vi "Circular.vi"(5 "Direction":u16(ring) items=["Clockwise", "Counter-clockwise"], 6 "return immediately":bool, 7 "Speed":dbl, 8 "error in (no error)":errorcluster, 9 "XY End":dbl[](array[numeric]), 10 "XY Center":dbl[](array[numeric]), 11 "Gantry":refnum<k24>) -> (0 "error IO":errorcluster, 3 "Gantry  2":refnum<k24>)   [LabVIEW 2020, in "Motion.lvclass"]
uses:
  Motion.lvclass
  C:/Program Files (x86)/Aerotech/A3200/LabVIEW/2010/Bin/Aerotech.A3200.dll
  Program Files (x86)/Aerotech/A3200/LabVIEW/2010/Bin/Aerotech.A3200.dll
  Drivers/Aerotech A3200/Motion/CircularCenter.vi
  Drivers/Aerotech A3200/Aerotech.lvlib
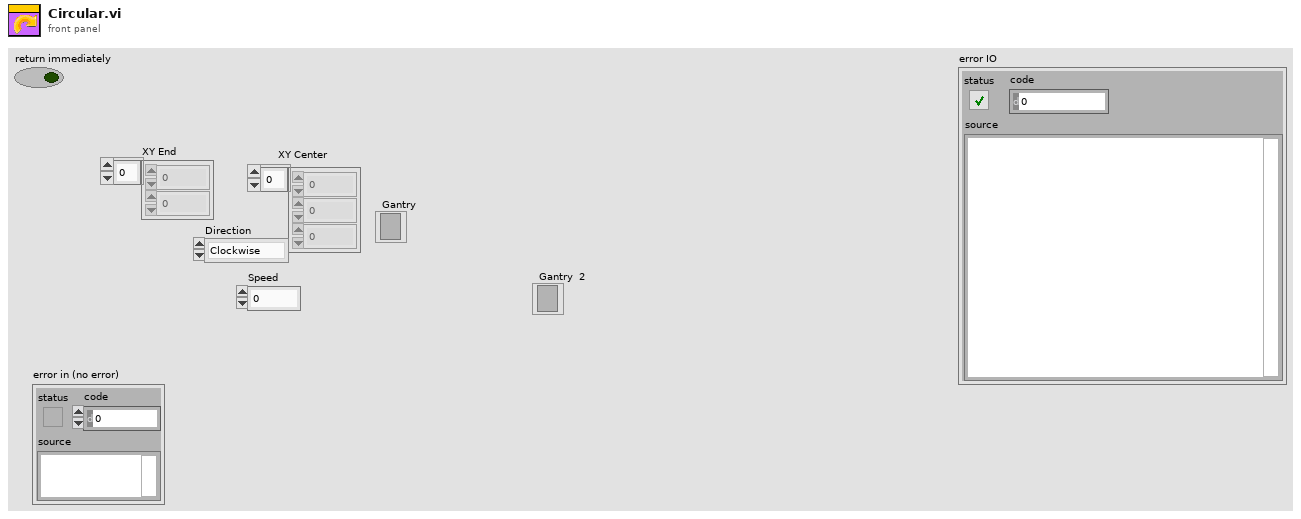
[diagram p1: front panel]
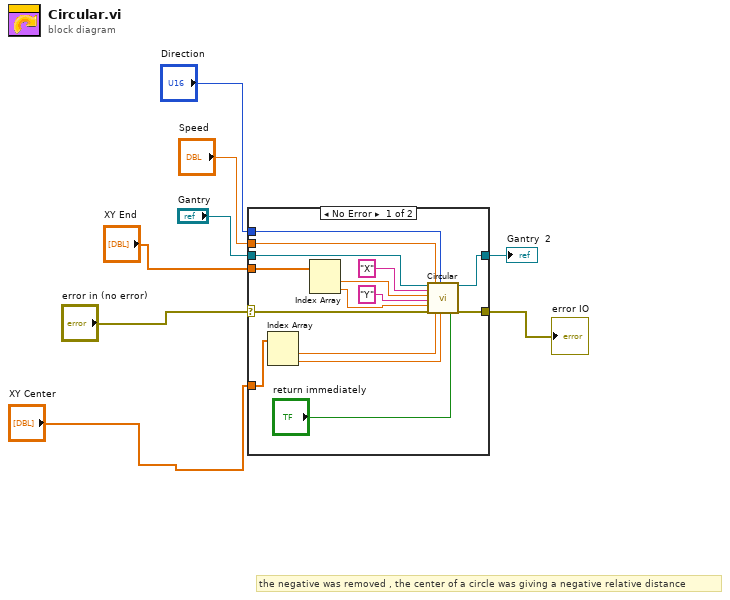
[diagram p0: block diagram]
diagram:
  # "the negative was removed , the center of a circle was giving a negative relative distance"
  n1 = case shown="No Error" "error in (no error)" {
    selector: "error in (no error)" -> [w17 w24]
    tunnel: "XY Center" -> [w22 _]
    tunnel: "Speed" -> [w16 _]
    tunnel: "Direction" -> [w23 _]
    tunnel: [w20 w25] -> w6
    tunnel: "Gantry" -> [w19 w25]
    tunnel: [w18 w24] -> w4
    tunnel: "XY End" -> [w9 _]
    frame No Error {
      n2 = Index Array(array=w22) -> (element #1=w11:dbl, element #2=w10:dbl)  [unwired: 2 in]
      n3 = Index Array(array=w9) -> (element #1=w14:dbl, element #2=w12:dbl)  [unwired: 2 in]
      n4 = call-poly "Circular.vi"("controller in"=w19, "axis 1 name"="X", "axis 1 endpoint"=w14, "axis 2 name"="Y", "axis 2 endpoint"=w12, "error in (no error)"=w17, "speed"=w16, "axis 1 center point"=w11, "direction"=w23, "axis 2 center point"=w10, "return immediately"="return immediately") -> ("controller out"=w20:refnum<k24>, "error out"=w18:errorcluster)  [unwired: 7 in]
    }
    frame Error {
    }
  }
  "Gantry  2" <- w6
  "error IO" <- w4
